vi "Check for Close.vi"(8 "error in":errorcluster, 11 "Peer Review":refnum<class "Peer Review.lvclass">) -> (0 "error out":errorcluster, 2 "Close?":bool)   [LabVIEW 2020, in "Peer Review.lvclass"]
uses:
  Peer Review.lvclass
  Peer Review.lvclass/Peer Review.ctl
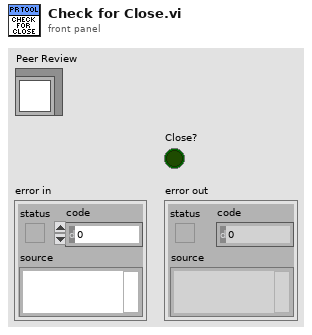
[diagram p1: front panel]
types:
  T1 = typedef "Peer Review.lvclass/File Info.ctl" = cluster{"File ID":i32, "Commit ID":i32, "Reviewed Hash":string, "Relative Path":string, "File Path":path, "File Checksum":string, "State":T2, "FP Changes":i32, "BD Changes":i32, "FP Bounds Error":dbl, "BD Bounds Error":dbl, "Lines Added":i32, "Lines Removed":i32, "Analysis Passes":i32, "Analysis Fails":i32, "Attribute Changes":i32, "Reentrancy State":string, "Cyclomatic Complexity":i32, "Node Count":i32, "Revision Number":u32, "LabVIEW Version":string, "Description":string, "Master Path":path, "Master Checksum":string, "VI Type":T3, "LabVIEW File":bool, "Review Complete":bool, "File Ref":refnum<vi>, "Master Revision":u32}
  T2 = typedef "Peer Review.lvclass/File State.ctl" = enum16{"Interrogation Needed", "Modified", "Deleted", "Added", "Matches Previous", "No Changes", "Moved", "Empty File"}
  T3 = typedef "Peer Review.lvclass/VI Type.ctl" = enum32{"invalid VI type", "Standard VI", "Control VI", "Global VI", "Polymorphic VI", "Configuration VI", "SubSystem", "Facade VI", "Method VI", "Statechart Diagram VI"}
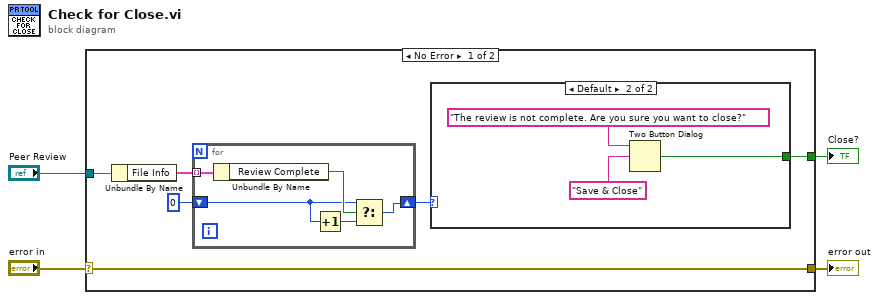
[diagram p0: block diagram]
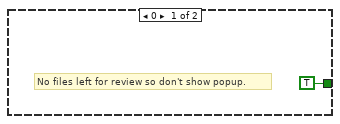
[diagram p2: hidden frame]
diagram:
  n1 = case shown="No Error" "error in" {
    selector: "error in" -> [w10 w20]
    tunnel: [w10 w20] -> w3
    tunnel: "Peer Review" -> [w7 _]
    tunnel: [w6 _] -> w1
    frame No Error {
      n2 = Unbundle By Name(w7) -> ("File Info"=w8:T1[])
      n3 = for {
        tunnel: w8 -> [w19] mode=indexing
        shift-right: [w15] -> w5
        shift-left: 0 -> [w16]
        n4 = Unbundle By Name(w19) -> ("Review Complete"=w18:bool)
        n5 = Increment(x=w16) -> (x+1=w17:i32)
        n6 = Select(t=w16, s=w18, f=w17) -> (s? t:f=w15:i32)
      }
      n7 = case shown="Default" w5 {
        tunnel: [TRUE ("T button?") w12] -> w6
        frame 0 {
          # "No files left for review so don't show popup."
        }
        frame Default {
          n8 = Two Button Dialog(message="The review is not complete. Are you sure you want to close?", 2:"Save & Close" ("T button name (\"OK\")")) -> (T button?=w12:bool)  [unwired: 1 in]
        }
      }
    }
    frame Error {
    }
  }
  "error out" <- w3
  "Close?" <- w1
